vi "Merge_into_Array.vi"(1 "Index":i32, 2 "Insert":i32, 3 "1D Array":i32[](array[numeric]), 4 "2D Array":i32[][](array[numeric])) -> (0 "Output Array":i32[][](array[numeric]))   [LabVIEW 2015]
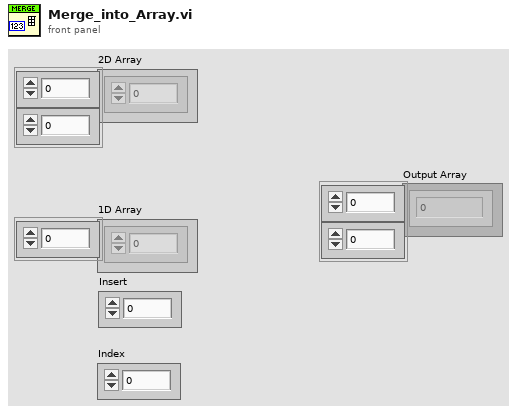
[diagram p1: front panel]
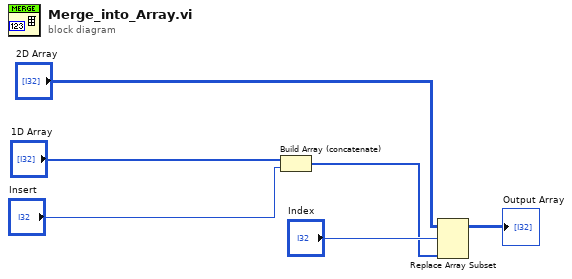
[diagram p0: block diagram]
diagram:
  n1 = Build Array (concatenate)("1D Array", "Insert") -> (w2:i32[])
  n2 = Replace Array Subset(array="2D Array", new element=w2, index (row)="Index") -> (→"Output Array":i32[][])  [unwired: 1 in]
